vi "Get Instrument Info.vi"(0 "Power Detector in":refnum<class "Power Detector.lvclass">, 11 "error in":errorcluster) -> (4 "Power Detector out":refnum<class "Power Detector.lvclass">, 15 "error out":errorcluster)   [LabVIEW 2023, in "NI CAL-5501 Power Detector.lvlib" / "Power Detector.lvclass"]
uses:
  Power Detector.lvclass
  C:/srd-semi-rfcal-software/AuxTools/STSRFFixtureCharactUtility/Source/Code Modules/Fixture/Instruments/Power Meter/Power Meter Base/Power Meter Base.lvclass
  Instruments/Power Meter/Power Meter Base/Type Definitions/Instrument Info.ctl
  Instruments/Power Meter/Power Meter Base/Power Meter Base.lvclass/Power Meter Base.ctl
  Instruments/Power Meter/Power Meter Base/Properties/Write Instrument Info Array.vi
  <vilib>/nisyscfg/Find Hardware.vi
  <vilib>/nisyscfg/Close (System).vi
  <resource>/objmgr/rfSysapiTags.rc
  <vilib>/nisyscfg/nisyscfg.lvlib
  Instruments/Power Meter/Power Meter Base/Power Meter Base.lvclass
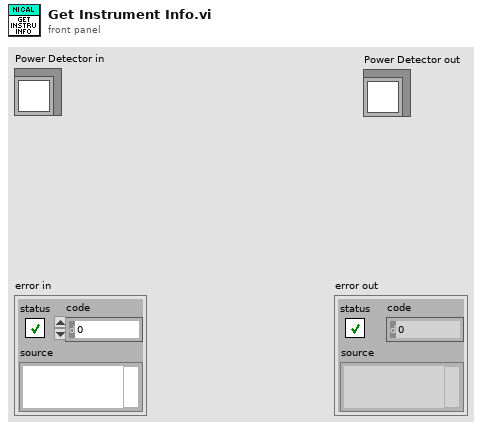
[diagram p1: front panel]
types:
  T1 = typedef "RFFixtureCharact.Instruments.lvlib/Power Meter Base.lvclass/Instrument Info.ctl" = cluster{"User Alias":string, "Resource Name":string, "Product Name":string, "Vendor Name":string}
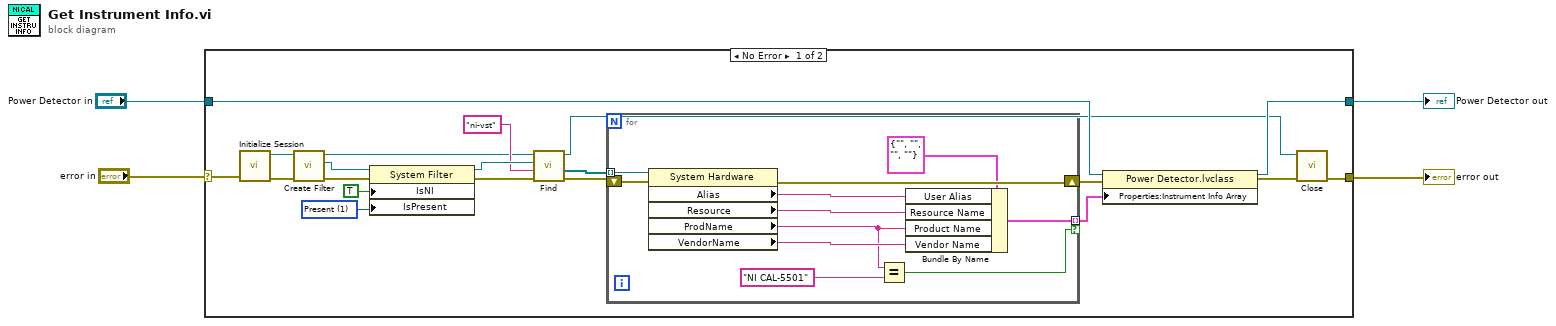
[diagram p0: block diagram]
diagram:
  n1 = case shown="No Error" "error in" {
    selector: "error in" -> [w15 w37]
    tunnel: [w11 w37] -> w2
    tunnel: "Power Detector in" -> [w8 w36]
    tunnel: [w7 w36] -> w3
    frame No Error {
      w14 = 1 items=["Unknown"=-1, "Not Present"=0, "Present"=1] ("Devices & Chassis:Is Present")
      n2 = call <vilib>:"Initialize Session.vi"("error in (no error)"=w15) -> ("error out"=w19:errorcluster, "Session out"=w21:refnum<k21>)  [unwired: 9 in]
      n3 = call <vilib>:"Create Filter.vi"("error in (no error)"=w19, "Session in"=w21) -> ("error out"=w24:errorcluster, "Filter out"=w16:refnum<k20>, "Session out"=w17:refnum<k21>)  [unwired: 7 in]
      n4 = property class="System Filter"(reference=w16, error in=w24, "IsNI"=TRUE ("Devices & Chassis:Is NI Product"), "IsPresent"=w14) -> (reference out=w23:refnum<k20>, error out=w22:errorcluster)
      n5 = call-poly <vilib>:"Find.vi"("error in (no error)"=w22, "Experts"="ni-vst", "Filter in"=w23, "Session in"=w17) -> ("error out"=w13:errorcluster, "Resources out"=w12:refnum<k20>[], "Session out"=w6:refnum<k21>)  [unwired: 4 in, 1 out]
      n6 = for {
        tunnel: w12 -> [w35] mode=indexing
        shift-right: [w34] -> w9
        shift-left: w13 -> [w33]
        tunnel: [w27] -> w5 mode=indexing if=w26
        n7 = property class="System Hardware"(reference=w35, error in=w33) -> (error out=w34:errorcluster, "Alias"=w30:string, "Resource"=w29:string, "ProdName"=w25:string, "VendorName"=w28:string)  [unwired: 1 out]
        n8 = Equal?(x=w25, y="NI CAL-5501") -> (x = y?=w26:bool)
        n9 = Bundle By Name(cluster=T1 {"User Alias"="", "Resource Name"="", "Product Name"="", "Vendor Name"=""} ("Instrument Info Cluster"), "User Alias"=w30, "Resource Name"=w29, "Product Name"=w25, "Vendor Name"=w28) -> (w27:T1)
      }
      n10 = property class="Power Detector.lvclass"(reference=w8, error in=w9, "Properties:Instrument Info Array"=w5) -> (reference out=w7:refnum<class "Power Detector.lvclass">, error out=w10:errorcluster)
      n11 = call-poly <vilib>:"Close.vi"("error in (no error)"=w10, "Session in"=w6) -> ("error out"=w11:errorcluster)  [unwired: 9 in]
    }
    frame Error {
    }
  }
  "error out" <- w2
  "Power Detector out" <- w3
